vi "Control_stage.vi"(8 "error in":errorcluster, 10 "Stage position IN":T1, 11 "Stage control IN":T2={"Up"=FALSE, "Left"=FALSE, "Right"=FALSE, "Down"=FALSE, "Z Down"=FALSE, "Z Up"=FALSE, "X Step Size(um)"=0.0, "Z step size (um)"=0.0, "Y Step Size(um)"=0.0, "Enable x-axis"=TRUE, "Enable y-axis"=TRUE, "Enable z-axis"=TRUE, "Same step size"=FALSE, "Global step size"=10.0, "stop"=FALSE}) -> (0 "error out":errorcluster, 2 "Stage position OUT":T1, 3 "Stage control OUT":T2={"Up"=FALSE, "Left"=FALSE, "Right"=FALSE, "Down"=FALSE, "Z Down"=FALSE, "Z Up"=FALSE, "X Step Size(um)"=0.0, "Z step size (um)"=0.0, "Y Step Size(um)"=0.0, "Enable x-axis"=TRUE, "Enable y-axis"=TRUE, "Enable z-axis"=TRUE, "Same step size"=FALSE, "Global step size"=10.0, "stop"=FALSE})   [LabVIEW 2020]
uses:
  typedefs/typedef_stage_control.ctl
  typedefs/typedef_stage_position.ctl
panel:
  out "Boolean 3":bool
  out "Boolean 2":bool
  out "Boolean":bool
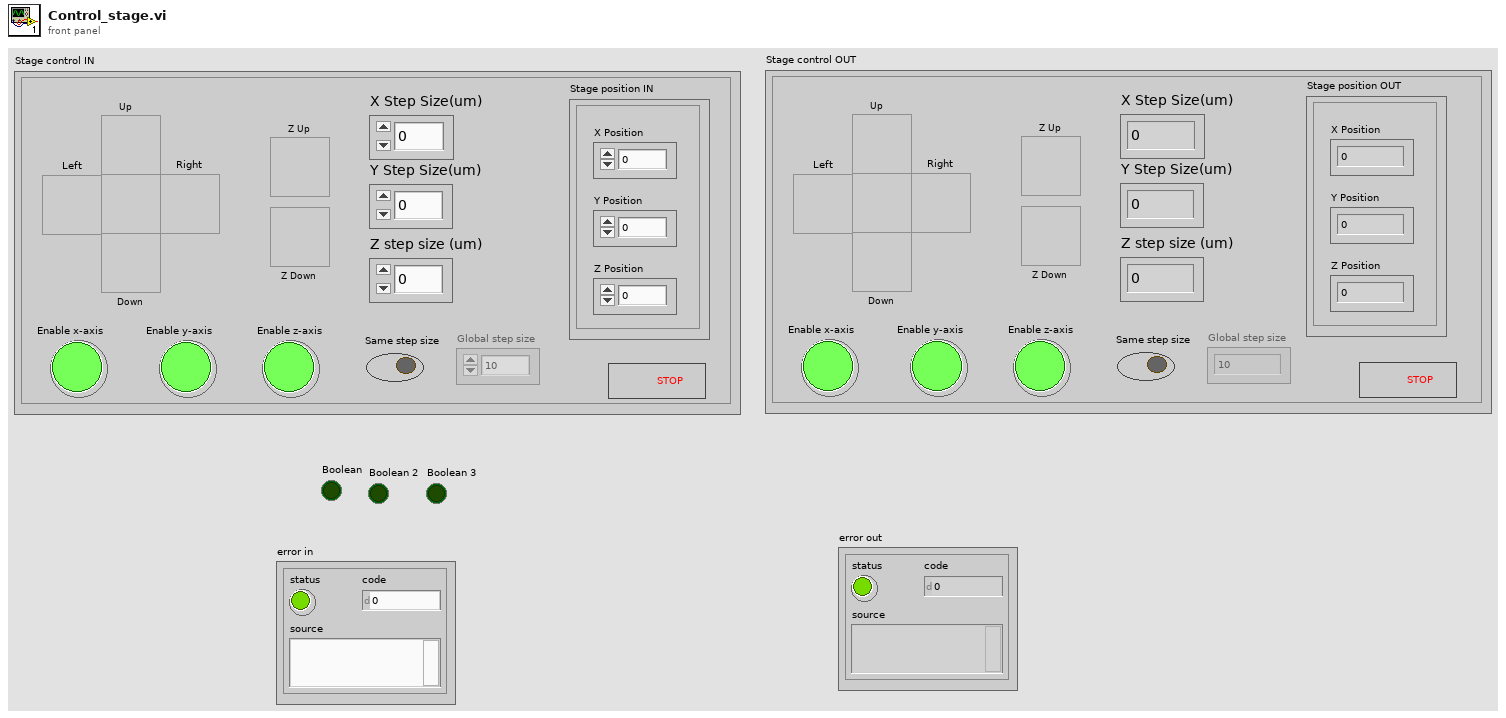
[diagram p1: front panel]
types:
  T1 = typedef "typedef_stage_position.ctl" = cluster{"X Position":dbl, "Y Position":dbl, "Z Position":dbl}
  T2 = typedef "typedef_stage_control.ctl" = cluster{"Up":bool, "Left":bool, "Right":bool, "Down":bool, "Z Down":bool, "Z Up":bool, "X Step Size(um)":dbl, "Z step size (um)":dbl, "Y Step Size(um)":dbl, "Enable x-axis":bool, "Enable y-axis":bool, "Enable z-axis":bool, "Same step size":bool, "Global step size":dbl, "stop":bool}
  T3 = enum8{"Enabled", "Disabled", "Disabled and Grayed Out"}
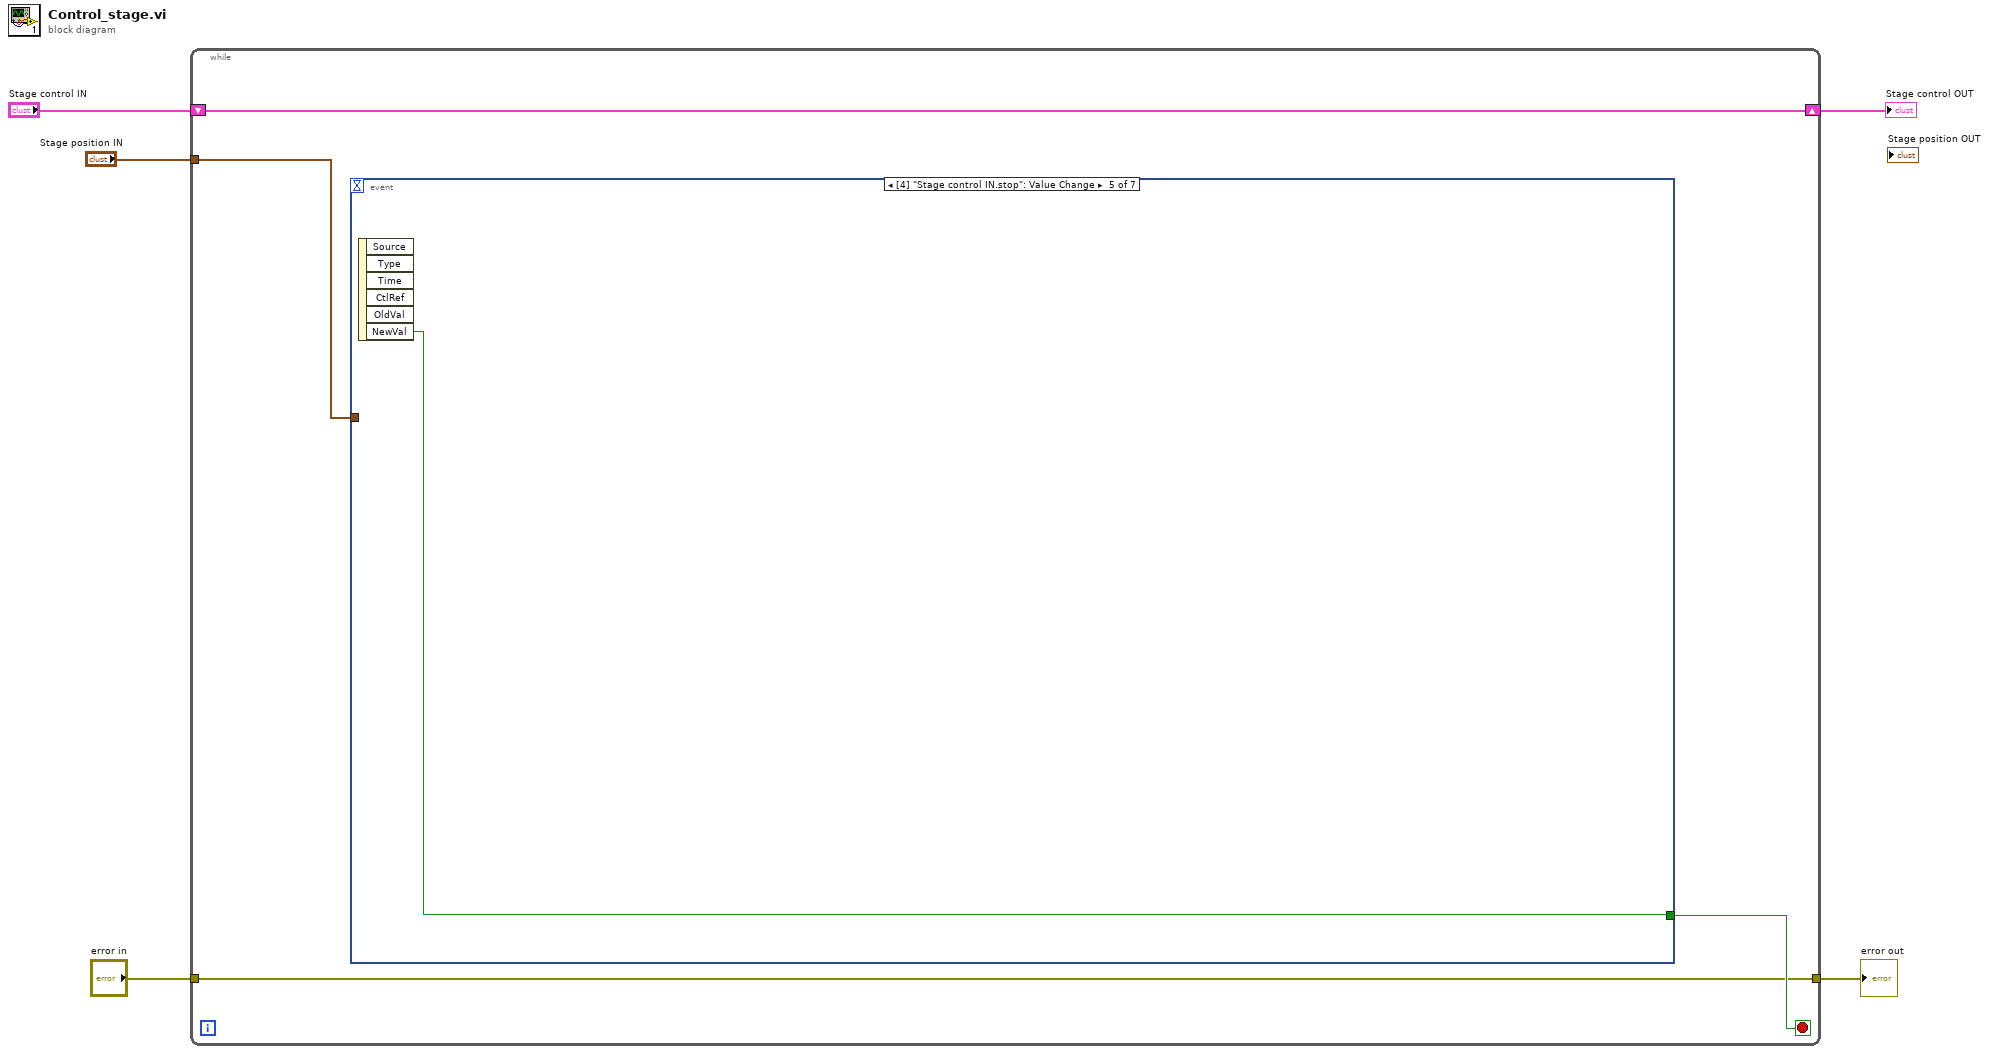
[diagram p0: block diagram]
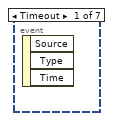
[diagram p2: hidden frame]
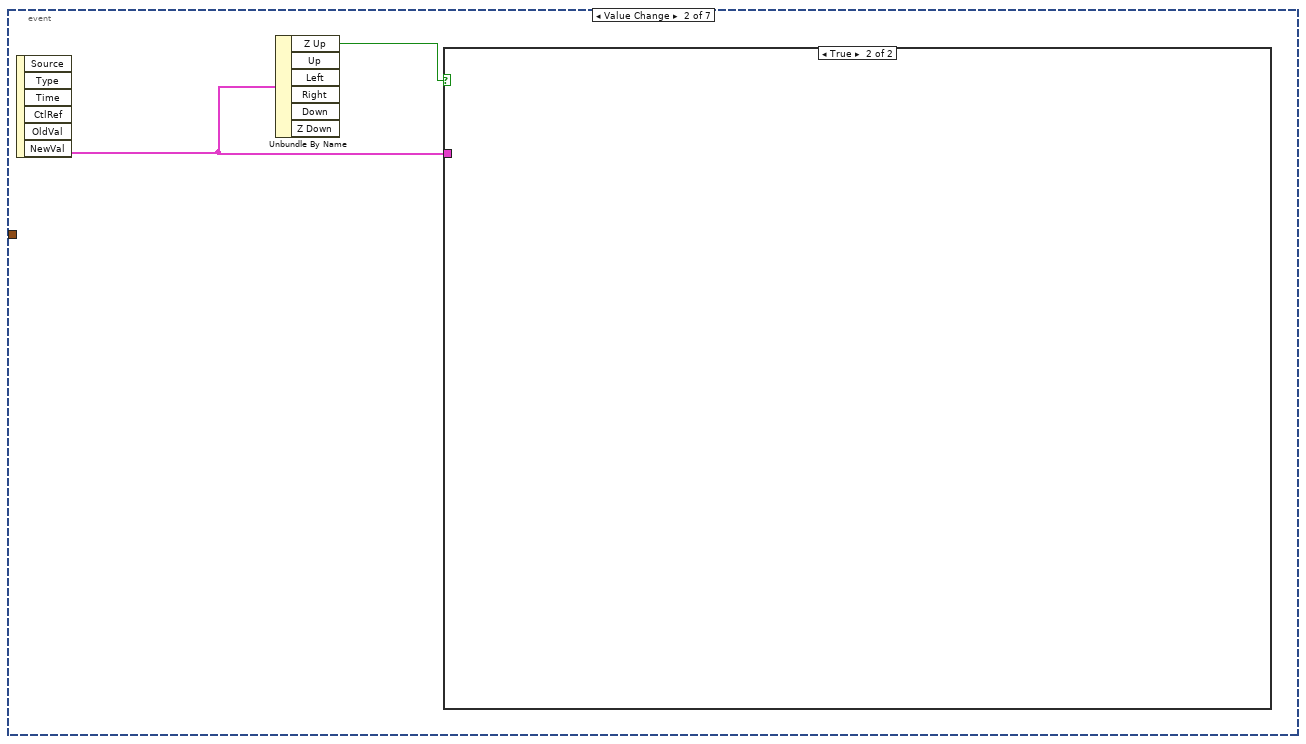
[diagram p3: hidden frame]
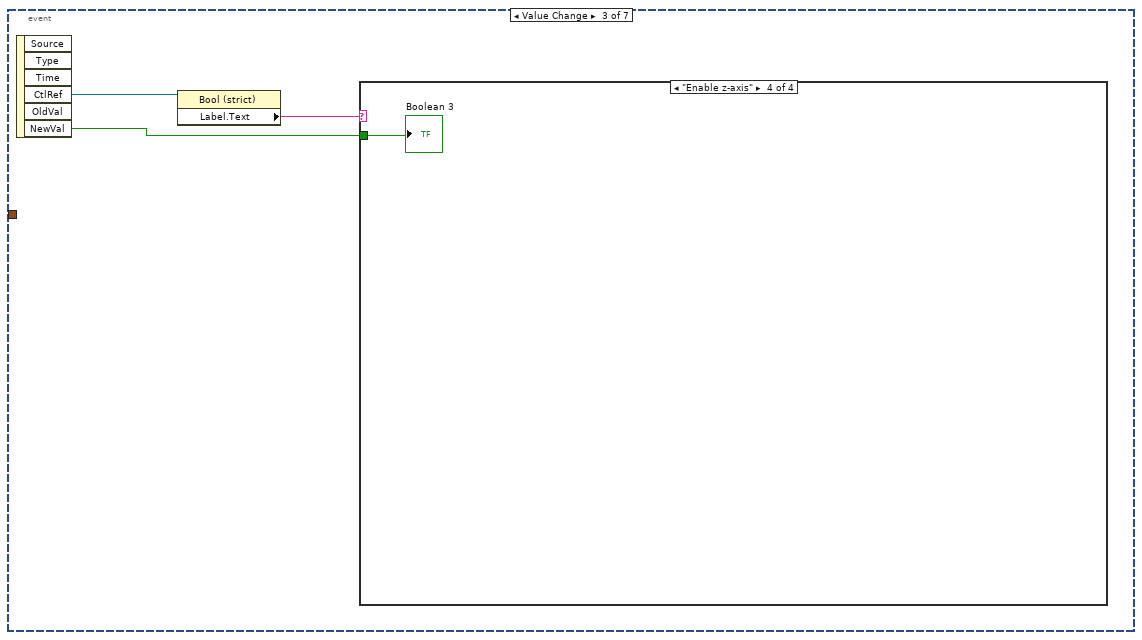
[diagram p5: hidden frame]
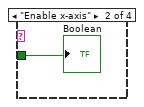
[diagram p7: hidden frame]
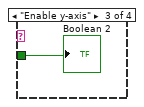
[diagram p8: hidden frame]
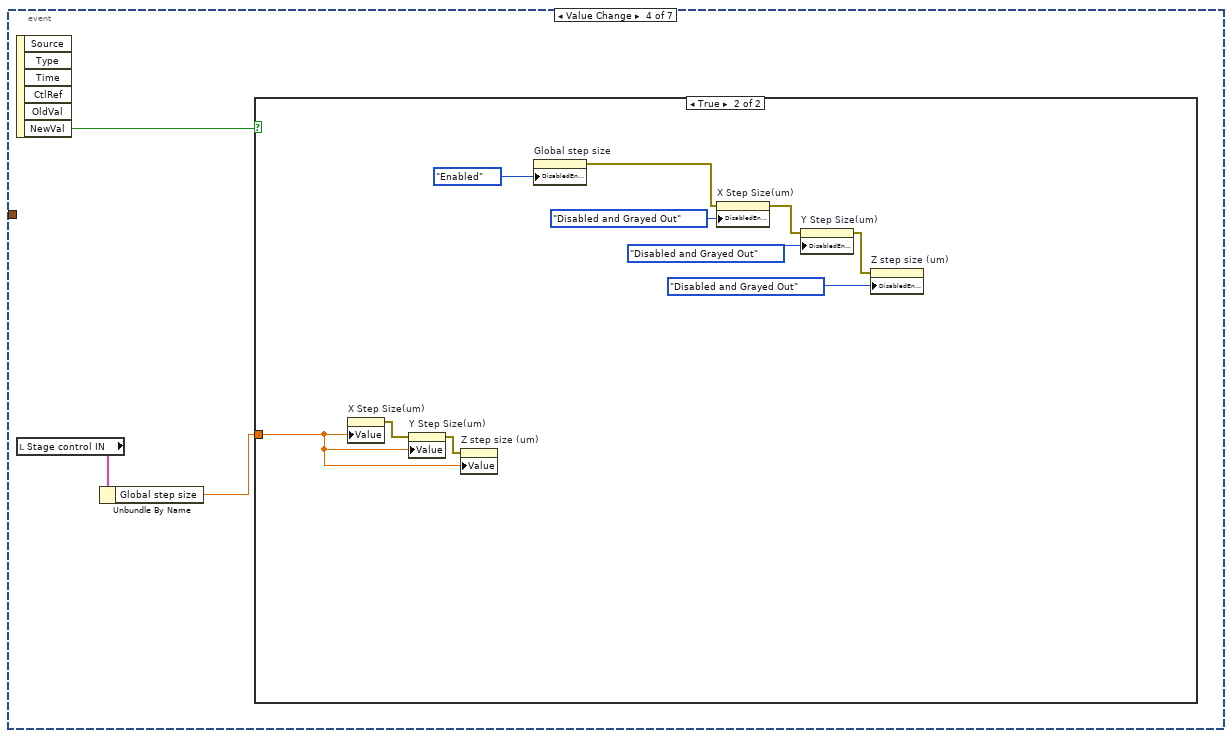
[diagram p9: hidden frame]
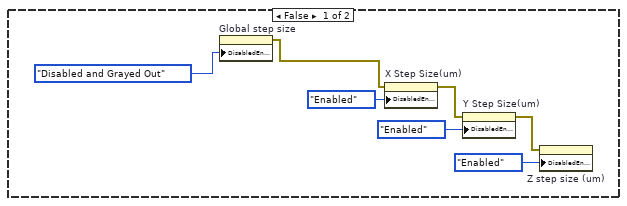
[diagram p10: hidden frame]
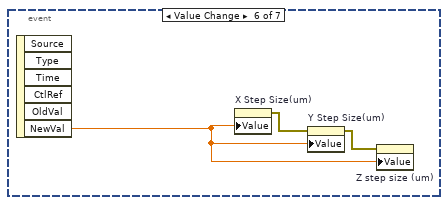
[diagram p11: hidden frame]
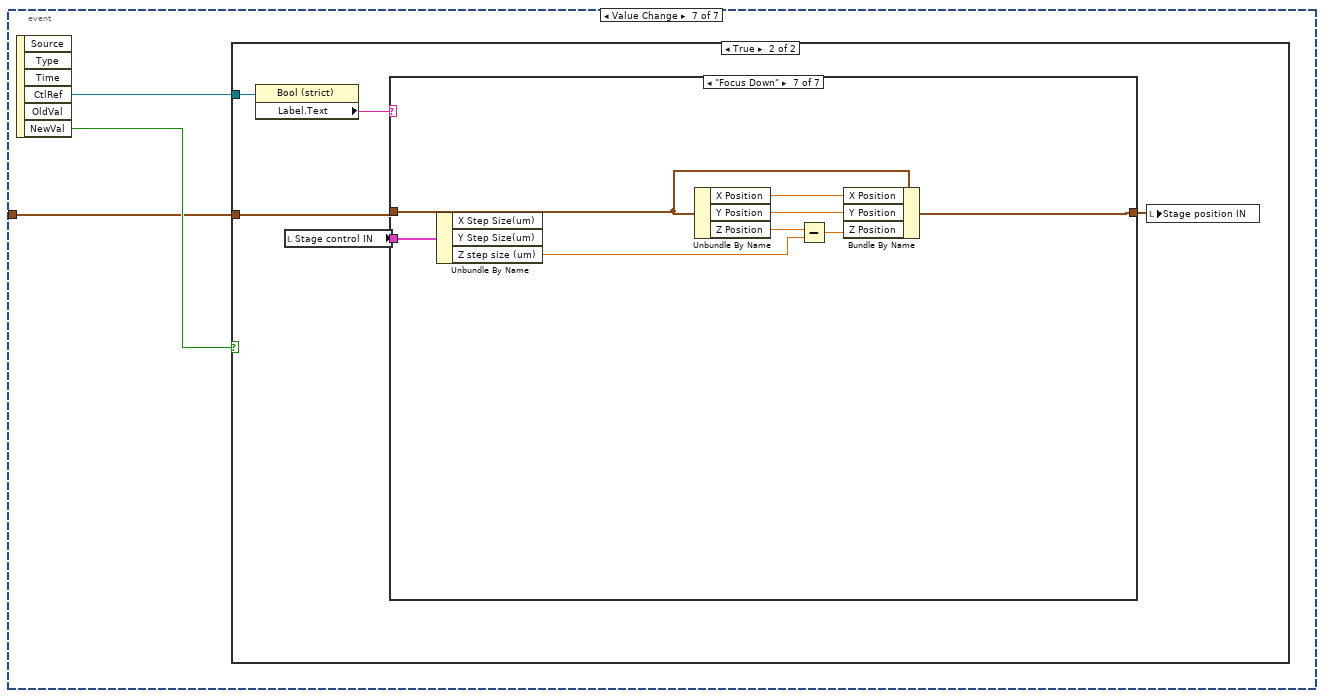
[diagram p12: hidden frame]
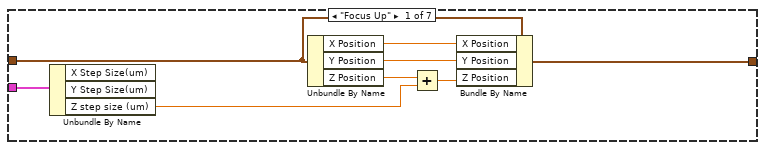
[diagram p14: hidden frame]
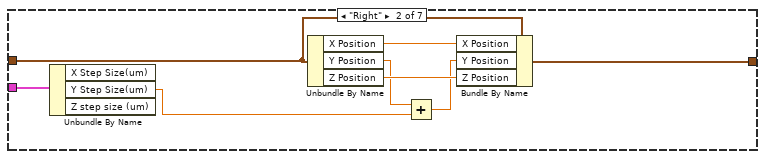
[diagram p15: hidden frame]
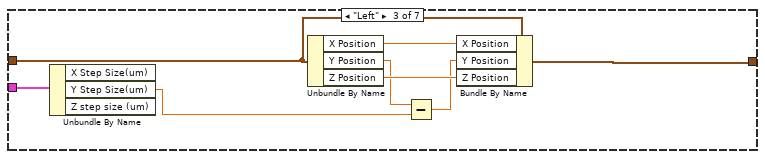
[diagram p16: hidden frame]
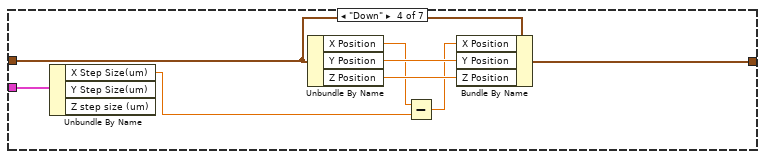
[diagram p17: hidden frame]
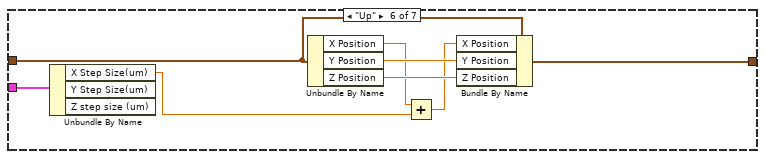
[diagram p19: hidden frame]
diagram:
  n1 = while {
    tunnel: "error in" -> [w8]
    tunnel: [w8] -> w4
    shift-right: [w7] -> w2
    shift-left: "Stage control IN" -> [w7]
    tunnel: "Stage position IN" -> [w6]
    stop <- w9 stop-if-true
    n2 = event shown="[4] \"Stage control IN.stop\": Value Change" {
      selector: _ -> [_ _ _ _ _ _ _]
      dyn-events: _ -> [_ _ _ _ _ _ _]
      timeout: _ -> [_ _ _ _ _ _ _]
      tunnel: [_ _ _ _ w38 _ _] -> w9
      tunnel: w6 -> [_ _ _ _ _ _ w42]
      event Timeout {
        n3 = event-data() -> ()  [unwired: 1 in, 3 out]
      }
      event Value Change {
        n4 = event-data() -> ("NewVal"=w11:T2)  [unwired: 1 in, 5 out]
        n5 = Unbundle By Name(w11) -> ("Z Up"=w10:bool)  [unwired: 5 out]
        n6 = case shown="True" w10 {
          tunnel: w11 -> [_ _]
          frame False {
          }
          frame True {
          }
        }
      }
      event Value Change {
        n7 = event-data() -> ("CtlRef"=w14:refnum<vi>, "NewVal"=w12:bool)  [unwired: 1 in, 4 out]
        n8 = property class="Bool (strict)"(reference=w14) -> ("Label.Text"=w13:string)  [unwired: 1 in, 2 out]
        n9 = case shown="\"Enable z-axis\"" w13 {
          tunnel: w12 -> [_ w15 w16 w17]
          frame Default {
          }
          frame "Enable x-axis" {
            "Boolean" <- w15
          }
          frame "Enable y-axis" {
            "Boolean 2" <- w16
          }
          frame "Enable z-axis" {
            "Boolean 3" <- w17
          }
        }
      }
      event Value Change {
        n10 = event-data() -> ("NewVal"=w20:bool)  [unwired: 1 in, 5 out]
        n11 = local read "Stage control IN"() -> (w19:T2)
        n12 = Unbundle By Name(w19) -> ("Global step size"=w18:dbl)
        n13 = case shown="True" w20 {
          tunnel: w18 -> [_ w32]
          frame False {
            n14 = property on="Global step size" class="DigNum (strict)"("DisabledEnum"=T3."Disabled and Grayed Out" ("Disabled")) -> (error out=w21:errorcluster)  [unwired: 2 in, 1 out]
            n15 = property on="X Step Size(um)" class="DigNum (strict)"(error in=w21, "DisabledEnum"=T3."Enabled" ("Disabled")) -> (error out=w25:errorcluster)  [unwired: 1 in, 1 out]
            n16 = property on="Y Step Size(um)" class="DigNum (strict)"(error in=w25, "DisabledEnum"=T3."Enabled" ("Disabled")) -> (error out=w23:errorcluster)  [unwired: 1 in, 1 out]
            n17 = property on="Z step size (um)" class="DigNum (strict)"(error in=w23, "DisabledEnum"=T3."Enabled" ("Disabled")) -> ()  [unwired: 1 in, 2 out]
          }
          frame True {
            n18 = property on="X Step Size(um)" class="DigNum (strict)"("Value"=w32) -> (error out=w31:errorcluster)  [unwired: 2 in, 1 out]
            n19 = property on="Y Step Size(um)" class="DigNum (strict)"(error in=w31, "Value"=w32) -> (error out=w30:errorcluster)  [unwired: 1 in, 1 out]
            n20 = property on="Z step size (um)" class="DigNum (strict)"(error in=w30, "Value"=w32) -> ()  [unwired: 1 in, 2 out]
            n21 = property on="Global step size" class="DigNum (strict)"("DisabledEnum"=T3."Enabled" ("Disabled")) -> (error out=w28:errorcluster)  [unwired: 2 in, 1 out]
            n22 = property on="X Step Size(um)" class="DigNum (strict)"(error in=w28, "DisabledEnum"=T3."Disabled and Grayed Out" ("Disabled")) -> (error out=w35:errorcluster)  [unwired: 1 in, 1 out]
            n23 = property on="Y Step Size(um)" class="DigNum (strict)"(error in=w35, "DisabledEnum"=T3."Disabled and Grayed Out" ("Disabled")) -> (error out=w33:errorcluster)  [unwired: 1 in, 1 out]
            n24 = property on="Z step size (um)" class="DigNum (strict)"(error in=w33, "DisabledEnum"=T3."Disabled and Grayed Out" ("Disabled")) -> ()  [unwired: 1 in, 2 out]
          }
        }
      }
      event Value Change {
        n25 = event-data() -> ("NewVal"=w38:bool)  [unwired: 1 in, 5 out]
      }
      event Value Change {
        n26 = event-data() -> ("NewVal"=w41:dbl)  [unwired: 1 in, 5 out]
        n27 = property on="X Step Size(um)" class="DigNum (strict)"("Value"=w41) -> (error out=w40:errorcluster)  [unwired: 2 in, 1 out]
        n28 = property on="Y Step Size(um)" class="DigNum (strict)"(error in=w40, "Value"=w41) -> (error out=w39:errorcluster)  [unwired: 1 in, 1 out]
        n29 = property on="Z step size (um)" class="DigNum (strict)"(error in=w39, "Value"=w41) -> ()  [unwired: 1 in, 2 out]
      }
      event Value Change {
        n30 = event-data() -> ("CtlRef"=w44:refnum<vi>, "NewVal"=w43:bool)  [unwired: 1 in, 4 out]
        n31 = case shown="True" w43 {
          tunnel: w44 -> [_ w49]
          tunnel: w42 -> [_ w45]
          frame False {
          }
          frame True {
            n32 = property class="Bool (strict)"(reference=w49) -> ("Label.Text"=w48:string)  [unwired: 1 in, 2 out]
            n33 = local read "Stage control IN"() -> (w47:T2)
            n34 = case shown="\"Focus Down\"" w48 {
              tunnel: w47 -> [w52 w63 w71 w80 _ w89 w95]
              tunnel: w45 -> [w53 w64 w72 w81 w82 w90 w93]
              tunnel: [w51 w59 w67 w75 w82 w84 w92] -> w46
              frame "Focus Up" {
                n35 = Unbundle By Name(w52) -> ("Z step size (um)"=w50:dbl)  [unwired: 2 out]
                n36 = Unbundle By Name(w53) -> ("X Position"=w56:dbl, "Y Position"=w55:dbl, "Z Position"=w54:dbl)
                n37 = Add(x=w54, y=w50) -> (x+y=w57:dbl)
                n38 = Bundle By Name(cluster=w53, "X Position"=w56, "Y Position"=w55, "Z Position"=w57) -> (w51:T1)
              }
              frame "Right" {
                n39 = Unbundle By Name(w63) -> ("Y Step Size(um)"=w58:dbl)  [unwired: 2 out]
                n40 = Unbundle By Name(w64) -> ("X Position"=w65:dbl, "Y Position"=w61:dbl, "Z Position"=w62:dbl)
                n41 = Add(x=w61, y=w58) -> (x+y=w60:dbl)
                n42 = Bundle By Name(cluster=w64, "X Position"=w65, "Y Position"=w60, "Z Position"=w62) -> (w59:T1)
              }
              frame "Left" {
                n43 = Unbundle By Name(w71) -> ("Y Step Size(um)"=w66:dbl)  [unwired: 2 out]
                n44 = Unbundle By Name(w72) -> ("X Position"=w73:dbl, "Y Position"=w69:dbl, "Z Position"=w70:dbl)
                n45 = Subtract(x=w69, y=w66) -> (x-y=w68:dbl)
                n46 = Bundle By Name(cluster=w72, "X Position"=w73, "Y Position"=w68, "Z Position"=w70) -> (w67:T1)
              }
              frame "Down" {
                n47 = Unbundle By Name(w80) -> ("X Step Size(um)"=w74:dbl)  [unwired: 2 out]
                n48 = Unbundle By Name(w81) -> ("X Position"=w77:dbl, "Y Position"=w78:dbl, "Z Position"=w79:dbl)
                n49 = Subtract(x=w77, y=w74) -> (x-y=w76:dbl)
                n50 = Bundle By Name(cluster=w81, "X Position"=w76, "Y Position"=w78, "Z Position"=w79) -> (w75:T1)
              }
              frame Default {
              }
              frame "Up" {
                n51 = Unbundle By Name(w89) -> ("X Step Size(um)"=w83:dbl)  [unwired: 2 out]
                n52 = Unbundle By Name(w90) -> ("X Position"=w86:dbl, "Y Position"=w87:dbl, "Z Position"=w88:dbl)
                n53 = Add(x=w86, y=w83) -> (x+y=w85:dbl)
                n54 = Bundle By Name(cluster=w90, "X Position"=w85, "Y Position"=w87, "Z Position"=w88) -> (w84:T1)
              }
              frame "Focus Down" {
                n55 = Unbundle By Name(w95) -> ("Z step size (um)"=w91:dbl)  [unwired: 2 out]
                n56 = Unbundle By Name(w93) -> ("X Position"=w97:dbl, "Y Position"=w96:dbl, "Z Position"=w94:dbl)
                n57 = Subtract(x=w94, y=w91) -> (x-y=w98:dbl)
                n58 = Bundle By Name(cluster=w93, "X Position"=w97, "Y Position"=w96, "Z Position"=w98) -> (w92:T1)
              }
            }
            n59 = local write "Stage position IN"(w46) -> ()
          }
        }
      }
    }
  }
  "error out" <- w4
  "Stage control OUT" <- w2
